vi "Configure Temperature (Thermistor).vi"(0 "VISA resource name":refnum<visa-resource-name>, 9 "Units (0: Celsius)":u16(ring) items=["Celsius", "Fahrenheit", "Kelvin"], 11 "error in (no error)":errorcluster) -> (4 "VISA resource name out":refnum<visa-resource-name>, 15 "error out":errorcluster)   [LabVIEW 2021, in "Agilent 34420.lvlib"]
doc: "Configures the units of measurement when using a thermistor for temperature measurements."
uses:
  <instrlib>/Agilent 34420/Agilent 34420.lvlib
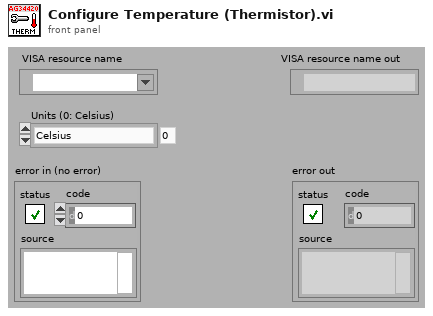
[diagram p1: front panel]
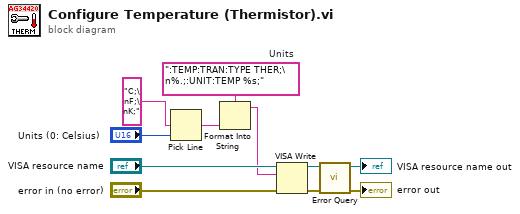
[diagram p0: block diagram]
diagram:
  w2 = ":TEMP:TRAN:TYPE THER;\n%.;:UNIT:TEMP %s;"  # Units
  n1 = Pick Line(multi-line string="C;\nF;\nK;", line index="Units (0: Celsius)") -> (output string=w3:string)  [unwired: 1 in]
  n2 = Format Into String(format string=w2, w3) -> (resulting string=w1:string)  [unwired: 2 in, 1 out]
  n3 = VISA Write(VISA resource name="VISA resource name", write buffer=w1, error in (no error)="error in (no error)") -> (VISA resource name out=w7:refnum<visa-resource-name>, error out=w6:errorcluster)  [unwired: 1 out]
  n4 = call <instrlib>:"Error Query.vi"("error in (no error)"=w6, "VISA resource name"=w7) -> ("error out"=→"error out":errorcluster, "VISA resource name out"=→"VISA resource name out":refnum<visa-resource-name>)  [unwired: 6 in, 2 out]
